vi "Estacionamiento.vi"() -> ()   [LabVIEW 2018]
panel:
  in  "Carro 3":bool
  in  "Carro 2":bool
  in  "Stop Button":bool
  in  "Carro 1":bool
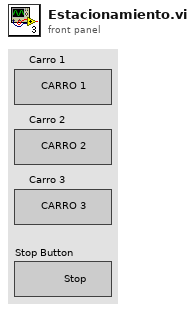
[diagram p1: front panel]
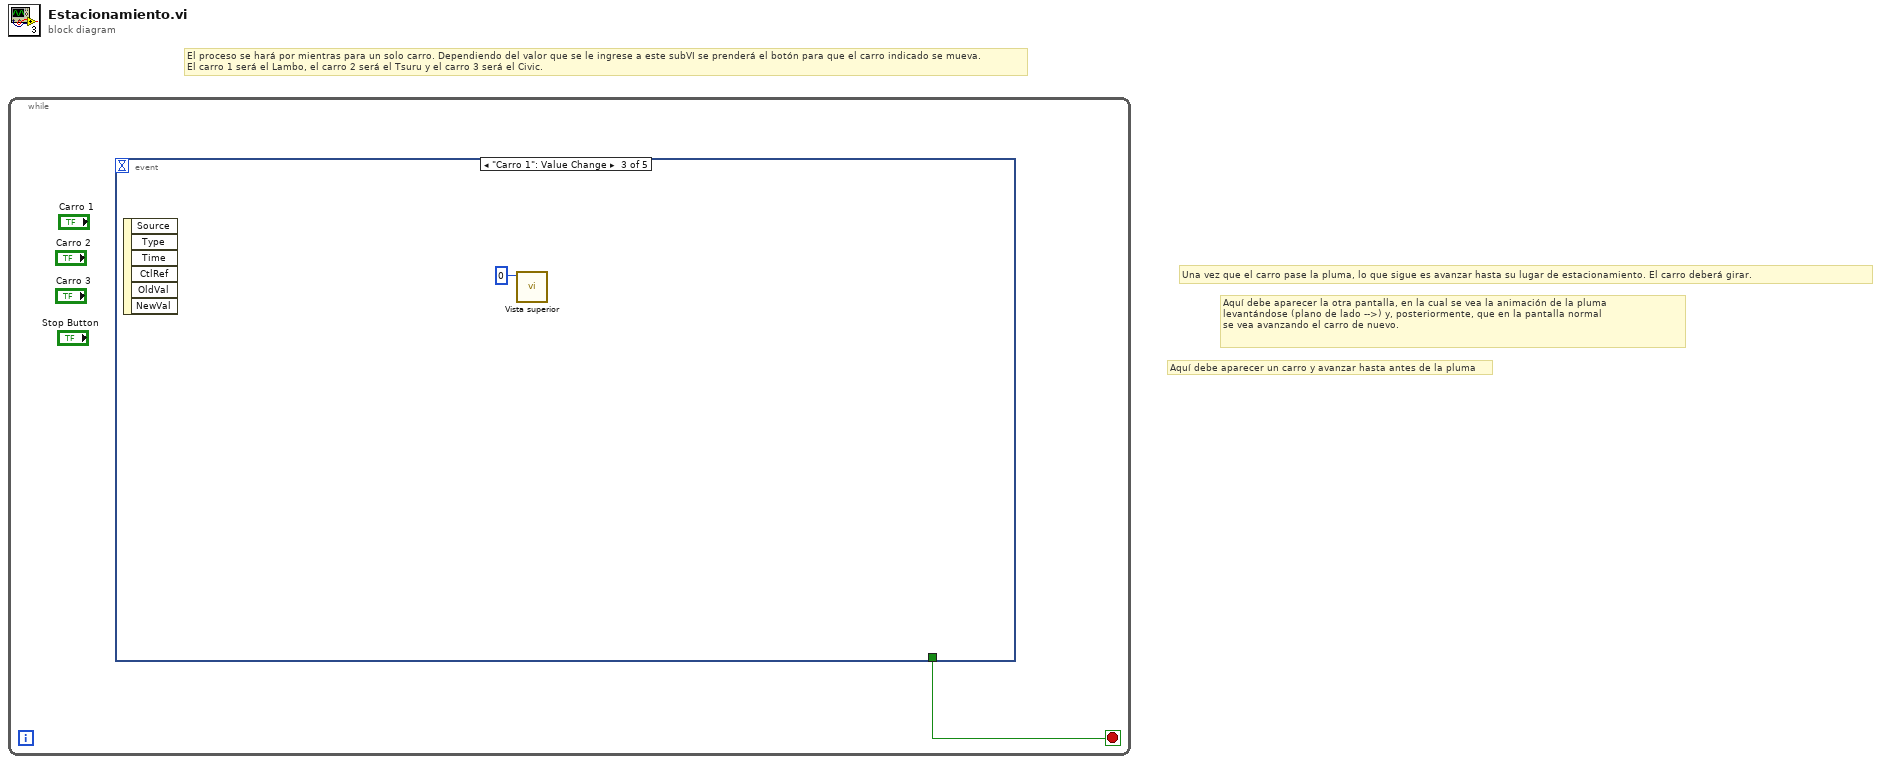
[diagram p0: block diagram]
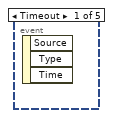
[diagram p2: hidden frame]
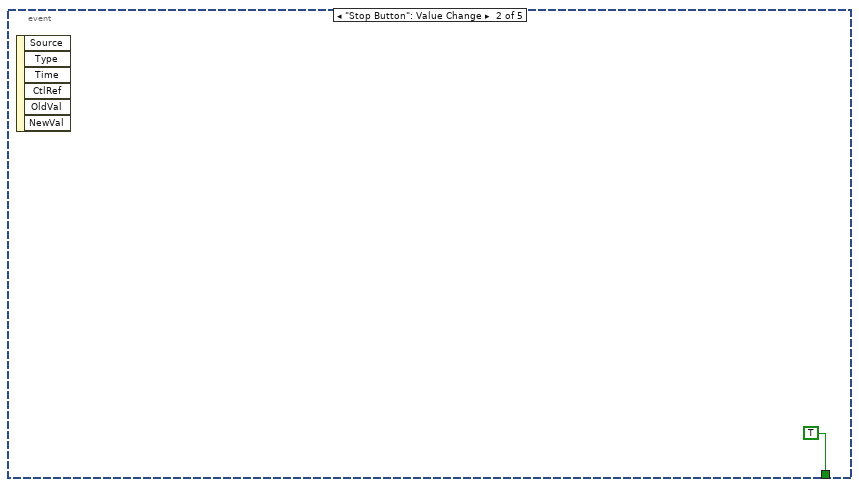
[diagram p3: hidden frame]
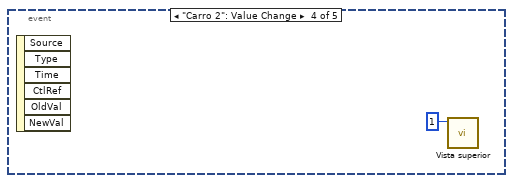
[diagram p4: hidden frame]
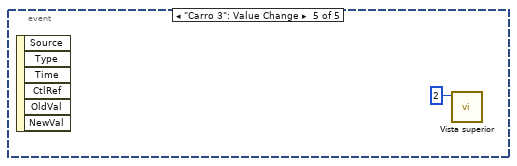
[diagram p5: hidden frame]
diagram:
  # "Una vez que el carro pase la pluma, lo que sigue es avanzar hasta su lugar de estacionamiento. El carro deberá girar."
  # "Aquí debe aparecer la otra pantalla, en la cual se vea la animación de la pluma\nlevantándose (plano de lado -->) y, posteriormente, que en la pantalla normal \nse vea avanzando el carro de nuevo."
  # "Aquí debe aparecer un carro y avanzar hasta antes de la pluma"
  # "El proceso se hará por mientras para un solo carro. Dependiendo del valor que se le ingrese a este subVI se prenderá el botón para que el carro indicado se mueva.\nEl carro 1 será el Lambo, el carro 2 será el Tsuru y el carro 3 será el Civic."
  n1 = while {
    stop <- w1 stop-if-true
    n2 = event shown="[2] \"Carro 1\": Value Change" {
      selector: _ -> [_ _ _ _ _]
      dyn-events: _ -> [_ _ _ _ _]
      timeout: _ -> [_ _ _ _ _]
      tunnel: [_ TRUE _ _ _] -> w1
      event Timeout {
        n3 = event-data() -> ()  [unwired: 1 in, 3 out]
      }
      event "Stop Button": Value Change {
        n4 = event-data() -> ()  [unwired: 1 in, 6 out]
      }
      event "Carro 1": Value Change {
        n5 = event-data() -> ()  [unwired: 1 in, 6 out]
        n6 = call "Vista superior.vi"("Numeric"=0) -> ()  [unwired: 11 in]
      }
      event "Carro 2": Value Change {
        n7 = event-data() -> ()  [unwired: 1 in, 6 out]
        n8 = call "Vista superior.vi"("Numeric"=1) -> ()  [unwired: 11 in]
      }
      event "Carro 3": Value Change {
        n9 = event-data() -> ()  [unwired: 1 in, 6 out]
        n10 = call "Vista superior.vi"("Numeric"=2) -> ()  [unwired: 11 in]
      }
    }
  }
